vi "Get OCT - Scaled Spectrums.vi"(0 "reference in":refnum<class "GSwFormDSP.lvclass">, 5 "error in (no error)":errorcluster, 6 "weighting":u16(ring) items=["Linear", "A-weighting", "B-weighting", "C-weighting"], 7 "Spectrums Display Options":T1(ring), 9 "Spectral Function Type":T2) -> (11 "Spectrum Unit":string[](array[string]), 13 "Octave Spectrums":waveform(dbl)[](array[waveform]), 14 "reference out":refnum<class "GSwFormDSP.lvclass">, 19 "error out":errorcluster)   [LabVIEW 2020, in "GSwFormDSP.lvclass"]
uses:
  GSwFormDSP.lvclass
  functions/Spectral Function Type.ctl
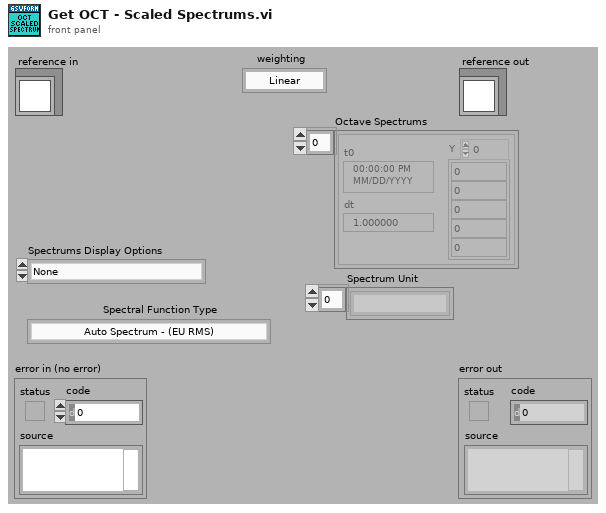
[diagram p1: front panel]
types:
  T1 = enum16{"None", "dB - NO reference value", "dB - Automatic reference value", "dB - Sound SPL (ref 20E-6 Pa)", "dB - Acceleration (ref 1E-6 m/s²)", "dB - Velocity (ref 1E-9 m/s)", "dB - Displacement (ref 1E-12 m)"}
  T2 = typedef "GSwFormDSP.lvclass/Spectral Function Type.ctl" = enum16{"Auto Spectrum - (EU RMS)", "Auto Spectrum - (EU Peak)", "Power Spectrum - (EU RMS²)", "Power Spectrum - (EU Peak²)", "Auto Spectrum Density - (EU RMS/rtHz)", "Auto Spectrum Density - (EU Peak/rtHz)", "Power Spectrum Density - (EU RMS²/Hz)", "Power Spectrum Density - (EU Peak²/Hz)"}
  T3 = cluster{"linear/dB":enum16{"no change", "linear", "dB"}, "dB reference (0: no change)":dbl, "power/magnitude":enum16{"no change", "power", "magnitude"}, "spectral density":enum16{"no change", "spectrum", "spectral density"}}
  T4 = enum16{"no change", "spectrum", "spectral density"}
  T5 = typedef "GSwFormDSP.lvclass/ObjectAttributes.ctl" = cluster{"Wform Ref":refnum<data-value>, "Nb Signals":i32, "Spectral Function Parameters":T6, "FFT":waveform(cdb)[], "Nb FFT":i32, "Nb Averages":i32[], "Reference Indexes":i32[], "Response Indexes":i32[], "Coherence":waveform(dbl)[], "TDF Parameters":T8, "DAQ":cluster{"Duration (sec)":dbl, "Buffer Size (Samples)":i32, "Offset (Samples)":i32}, "Filter Impulse Response (TDF)":waveform(dbl), "Sound Playback":T9}
  T6 = typedef "GSwFormDSP.lvclass/Spectral Parameters.ctl" = cluster{"Frequency resolution (Hz)":dbl, "Overlap":dbl, "Window":T7}
  T7 = typedef "NI_AALPro.lvlib/windowTd.ctl" = u32
  T8 = typedef "GSwFormDSP.lvclass/TDF Parameters.ctl" = cluster{"Filter":enum32{"Lowpass", "Highpass", "Bandpass", "Bandstop"}, "Type:":enum16{"Butterworth", "Chebyshev", "Inv Chebyshev", "Elliptic", "Bessel"}, "LP cutoff freq":dbl, "HP cutoff freq":dbl, "Order":i32, "passband ripple (dB)":dbl, "stopband attenuation (dB)":dbl, "Phaseless Filter":bool, "Include Fade IN and OUT":bool}
  T9 = typedef "GSwFormDSP.lvclass/Sound Playback.ctl" = cluster{"Timer start (ms)":u32, "task ID":T10, "Cursor Init Location (s)":dbl, "SC Volume":dbl}
  T10 = typedef "Sound Output Task ID.ctl" = u32
  T11 = enum16{"1 octave", "1/3 octave", "1/6 octave", "1/12 octave", "1/24 octave"}
  T12 = cluster{"nominal frequencies [Hz]":dbl[], "band power":dbl[]}[]
  T13 = typedef "SoundVib_Octave.lvlib/sv_Octave Info.ctl" = cluster{"standard":enum16{"ANSI S.1.11", "IEC 1260"}, "bandwidth":enum16{"1 octave", "1/3 octave", "1/6 octave", "1/12 octave", "1/24 octave"}, "low band":i32, "high band":i32, "weighting filter":T14, "dB reference":dbl, "dB On":bool, "unit label":string, "channel name":string, "description":string, "engineering units":T15, "custom label":string, "spectrum type":enum16{"power", "magnitude"}, "spectral density":bool, "filters settled":bool}
  T14 = typedef "svc_Weighting Filter Text Ring.ctl" = u16
  T15 = typedef "svc_Engineering Units Text Ring.ctl" = u16
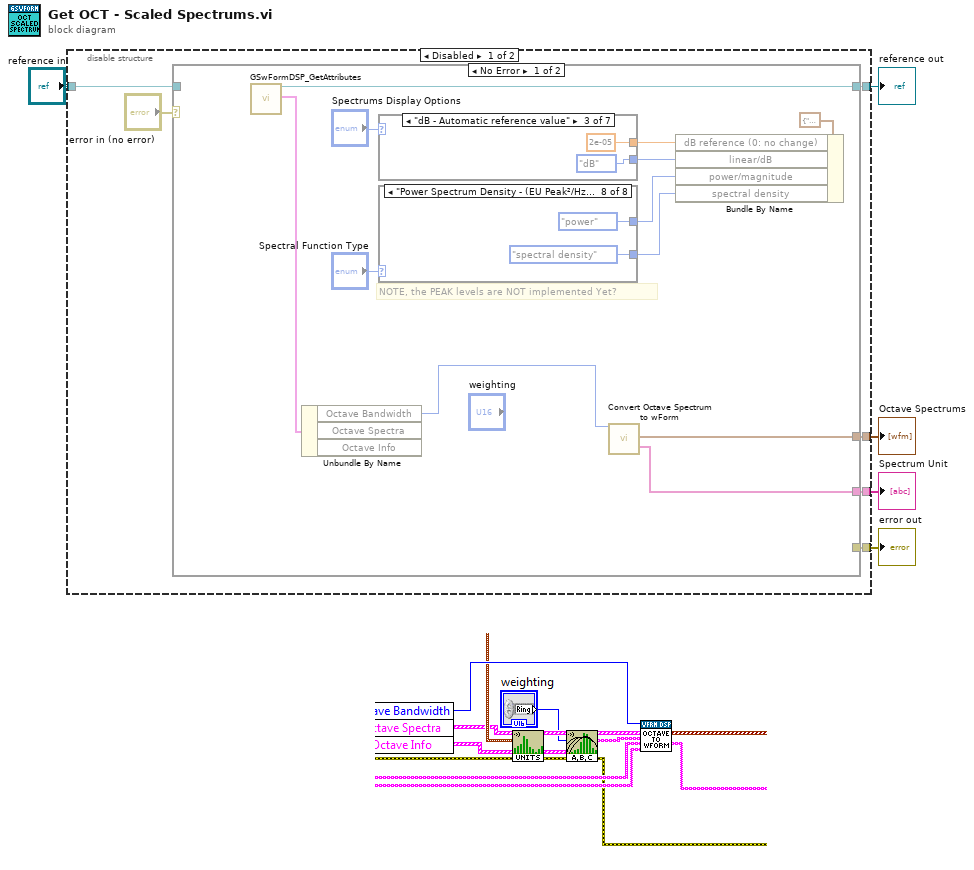
[diagram p0: block diagram]
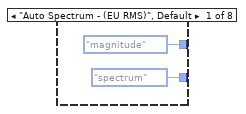
[diagram p2: hidden frame]
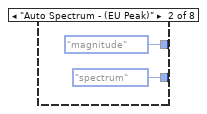
[diagram p3: hidden frame]
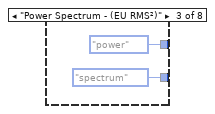
[diagram p4: hidden frame]
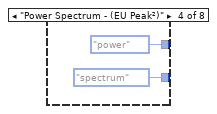
[diagram p5: hidden frame]
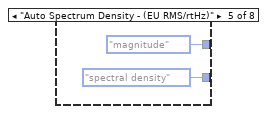
[diagram p6: hidden frame]
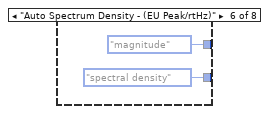
[diagram p7: hidden frame]
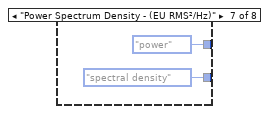
[diagram p8: hidden frame]
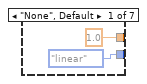
[diagram p9: hidden frame]
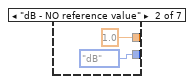
[diagram p10: hidden frame]
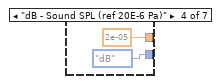
[diagram p11: hidden frame]
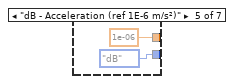
[diagram p12: hidden frame]
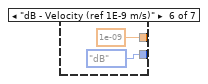
[diagram p13: hidden frame]
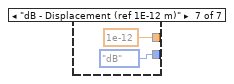
[diagram p14: hidden frame]
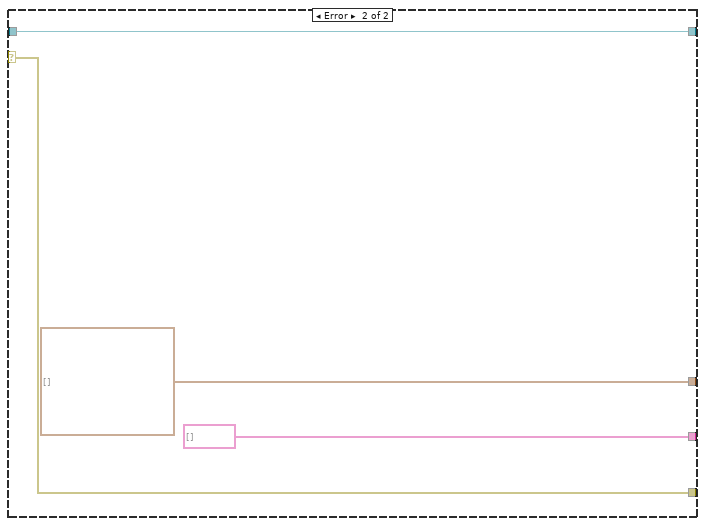
[diagram p15: hidden frame]
diagram:
  n1 = disable-structure shown="Disabled" {
    disable-tunnel: [w10 _] -> w5
    disable-tunnel: "reference in" -> [w9 _]
    disable-tunnel: [w8 _] -> w3
    disable-tunnel: [w7 _] -> w2
    disable-tunnel: [w6 _] -> w1
    frame Disabled {
      n2 = case shown="No Error" "error in (no error)" {
        selector: "error in (no error)" -> [_ w66]
        tunnel: [w18 w66] -> w10
        tunnel: [w32 w65] -> w8
        tunnel: w9 -> [_ w65]
        tunnel: [w12 waveform(dbl)[] []] -> w7
        tunnel: [w13 string[] []] -> w6
        frame No Error {
          # "NOTE, the PEAK levels are NOT implemented Yet?"
          n3 = call "GSwFormDSP_GetAttributes.vi"() -> ("reference out"=w32:refnum<class "GSwFormDSP.lvclass">, "attributes"=w31:T5, "error out"=w27:errorcluster)  [unwired: 16 in, 1 out]
          n4 = Unbundle By Name(w31) -> ("Octave Bandwidth"=w17:T11, "Octave Spectra"=w29:T12, "Octave Info"=w28:T13[])
          n5 = case shown="\"dB - Automatic reference value\"" "Spectrums Display Options" {
            tunnel: [1.0 ("dB reference (0: no change)") 1.0 ("dB reference (0: no change)") 2e-05 ("dB reference (0: no change)") 2e-05 ("dB reference (0: no change)") 1e-06 ("dB reference (0: no change)") 1e-09 ("dB reference (0: no change)") 1e-12 ("dB reference (0: no change)")] -> w24
            tunnel: [enum16{"no change", "linear", "dB"}."linear" ("linear/dB") enum16{"no change", "linear", "dB"}."dB" ("linear/dB") enum16{"no change", "linear", "dB"}."dB" ("linear/dB") enum16{"no change", "linear", "dB"}."dB" ("linear/dB") enum16{"no change", "linear", "dB"}."dB" ("linear/dB") enum16{"no change", "linear", "dB"}."dB" ("linear/dB") enum16{"no change", "linear", "dB"}."dB" ("linear/dB")] -> w23
            frame "None", Default {
            }
            frame "dB - NO reference value" {
            }
            frame "dB - Automatic reference value" {
            }
            frame "dB - Sound SPL (ref 20E-6 Pa)" {
            }
            frame "dB - Acceleration (ref 1E-6 m/s²)" {
            }
            frame "dB - Velocity (ref 1E-9 m/s)" {
            }
            frame "dB - Displacement (ref 1E-12 m)" {
            }
          }
          n6 = case shown="\"Power Spectrum Density - (EU Peak²/Hz)\"" "Spectral Function Type" {
            tunnel: [enum16{"no change", "power", "magnitude"}."magnitude" ("power/magnitude") enum16{"no change", "power", "magnitude"}."magnitude" ("power/magnitude") enum16{"no change", "power", "magnitude"}."power" ("power/magnitude") enum16{"no change", "power", "magnitude"}."power" ("power/magnitude") enum16{"no change", "power", "magnitude"}."magnitude" ("power/magnitude") enum16{"no change", "power", "magnitude"}."magnitude" ("power/magnitude") enum16{"no change", "power", "magnitude"}."power" ("power/magnitude") enum16{"no change", "power", "magnitude"}."power" ("power/magnitude")] -> w20
            tunnel: [T4."spectrum" ("spectral density") T4."spectrum" ("spectral density") T4."spectrum" ("spectral density") T4."spectrum" ("spectral density") T4."spectral density" ("spectral density") T4."spectral density" ("spectral density") T4."spectral density" ("spectral density") T4."spectral density" ("spectral density")] -> w19
            frame "Auto Spectrum - (EU RMS)", Default {
            }
            frame "Auto Spectrum - (EU Peak)" {
            }
            frame "Power Spectrum - (EU RMS²)" {
            }
            frame "Power Spectrum - (EU Peak²)" {
            }
            frame "Auto Spectrum Density - (EU RMS/rtHz)" {
            }
            frame "Auto Spectrum Density - (EU Peak/rtHz)" {
            }
            frame "Power Spectrum Density - (EU RMS²/Hz)" {
            }
            frame "Power Spectrum Density - (EU Peak²/Hz)" {
            }
          }
          n7 = call "Convert Octave Spectrum to wForm.vi"("Octave Bandwidth"=w17) -> ("octave spectra"=w16:T12, "Signal Names"=w15:string[], "Signal Units"=w14:string[], "wForm"=w12:waveform(dbl)[], "Units OUT"=w13:string[])  [unwired: 14 in]
          n8 = Bundle By Name(cluster=T3 {"linear/dB"=enum."no change", "dB reference (0: no change)"=0.0, "power/magnitude"=enum."no change", "spectral density"=enum."no change"} ("desired scaling"), "dB reference (0: no change)"=w24, "linear/dB"=w23, "power/magnitude"=w20, "spectral density"=w19) -> (w22:T3)
        }
        frame Error {
        }
      }
    }
    frame Enabled {
    }
  }
  "error out" <- w5
  "reference out" <- w3
  "Octave Spectrums" <- w2
  "Spectrum Unit" <- w1
